vi "Read SubDataEvents.vi"(11 "UserEvents in":refnum<class "UserEvents.lvclass">) -> (2 "SubDataEvents":T1, 3 "UserEvents out":refnum<class "UserEvents.lvclass">)   [LabVIEW 2013, in "UserEvents.lvclass"]
uses:
  UserEvents.lvclass
  Typedefs/SubDataEvents.ctl
  UserEvents.lvclass/UserEvents.ctl
  Typedefs/FAMTTypedefs.lvlib
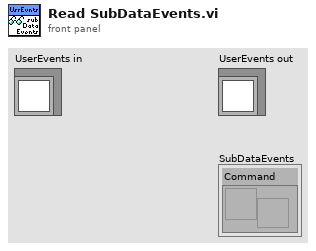
[diagram p1: front panel]
types:
  T1 = typedef "FAMTTypedefs.lvlib/SubDataEvents.ctl" = cluster{"Command":refnum<user-event>}
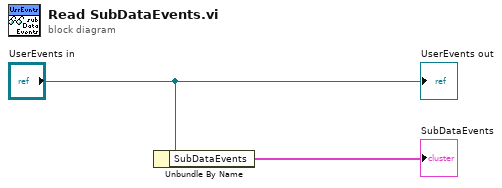
[diagram p0: block diagram]
diagram:
  n1 = Unbundle By Name("UserEvents in") -> ("SubDataEvents"=→"SubDataEvents":T1)
  "UserEvents out" <- "UserEvents in"
